vi "Queued Pedestrian Lights.vi"() -> ()   [LabVIEW 2012]
doc: "Traffic Light VI with the use of Queues. Has control over both the Traffic Lights Display and the Pedestrian Lights Display. Red is set as the initial State."
uses:
  Controls/Traffic Light Display.ctl
  Controls/Pedestrian Light Display.ctl
  Controls/Traffic Light States (with Walk State).ctl
panel:
  out "Pedestrian Light Display":T1
  in  "Walk":bool
  in  "Stop Button":bool
  out "Traffic Light Display":T2
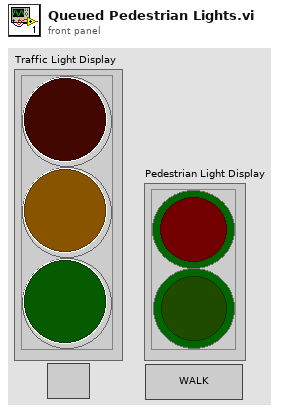
[diagram p1: front panel]
types:
  T1 = typedef "Pedestrian Light Display.ctl" = cluster{"Red":bool, "Green":bool}
  T2 = typedef "Traffic Light Display.ctl" = cluster{"RED":bool, "AMBER":bool, "GREEN":bool}
  T3 = typedef "Traffic Light States (with Walk State).ctl" = enum16{"Red", "RedAmber", "Green", "Amber", "Walk"}
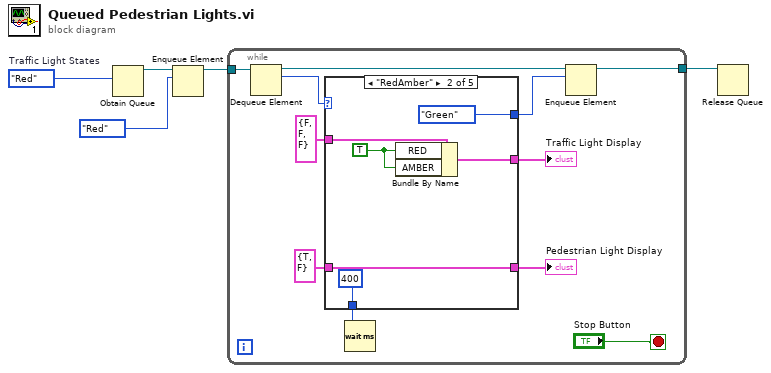
[diagram p0: block diagram]
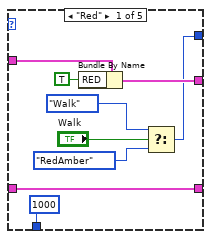
[diagram p2: hidden frame]
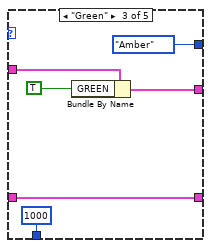
[diagram p3: hidden frame]
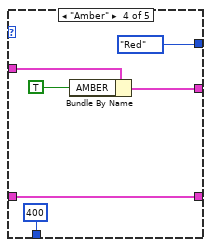
[diagram p4: hidden frame]
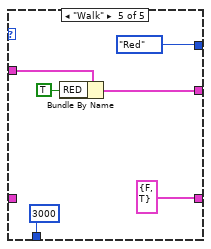
[diagram p5: hidden frame]
diagram:
  w2 = Traffic_Light_States_(with_Walk_State)."Red"  # Traffic Light States
  n1 = Obtain Queue(element data type=w2) -> (queue out=w5:refnum<queue>)  [unwired: 4 in, 2 out]
  n2 = Enqueue Element(queue=w5, element=Traffic_Light_States_(with_Walk_State)."Red") -> (queue out=w4:refnum<queue>)  [unwired: 2 in, 2 out]
  n3 = while {
    tunnel: w4 -> [w10]
    tunnel: [w6] -> w3
    stop <- "Stop Button" stop-if-true
    n4 = Dequeue Element(queue=w10) -> (queue out=w7:refnum<queue>, element=w9:T3)  [unwired: 2 in, 2 out]
    n5 = case shown="\"RedAmber\"" w9 {
      tunnel: T2 {"RED"=FALSE, "AMBER"=FALSE, "GREEN"=FALSE} ("Traffic Light Display") -> [w25 w31 w37 w43 w48]
      tunnel: [w23 w30 w35 w41 w46] -> w15
      tunnel: [w20 Traffic_Light_States_(with_Walk_State)."Green" Traffic_Light_States_(with_Walk_State)."Amber" Traffic_Light_States_(with_Walk_State)."Red" Traffic_Light_States_(with_Walk_State)."Red"] -> w8
      tunnel: [1000 400 1000 400 3000] -> w13
      tunnel: T1 {"Red"=TRUE, "Green"=FALSE} ("Pedestrian Light Display") -> [w19 w27 w33 w39 _]
      tunnel: [w19 w27 w33 w39 T1 {"Red"=FALSE, "Green"=TRUE} ("Pedestrian Light Display")] -> w11
      frame "Red" {
        n6 = Bundle By Name(cluster=w25, "RED"=TRUE) -> (w23:T2)
        n7 = Select(t=Traffic_Light_States_(with_Walk_State)."Walk", s="Walk", f=Traffic_Light_States_(with_Walk_State)."RedAmber") -> (s? t:f=w20:T3)
      }
      frame "RedAmber" {
        w29 = TRUE ("RED")
        n8 = Bundle By Name(cluster=w31, "RED"=w29, "AMBER"=w29) -> (w30:T2)
      }
      frame "Green" {
        n9 = Bundle By Name(cluster=w37, "GREEN"=TRUE ("RED")) -> (w35:T2)
      }
      frame "Amber" {
        n10 = Bundle By Name(cluster=w43, "AMBER"=TRUE ("RED")) -> (w41:T2)
      }
      frame "Walk" {
        n11 = Bundle By Name(cluster=w48, "RED"=TRUE) -> (w46:T2)
      }
    }
    "Traffic Light Display" <- w15
    "Pedestrian Light Display" <- w11
    n12 = Wait (ms)(milliseconds to wait=w13) -> ()  [unwired: 1 out]
    n13 = Enqueue Element(queue=w7, element=w8) -> (queue out=w6:refnum<queue>)  [unwired: 2 in, 2 out]
  }
  n14 = Release Queue(queue=w3) -> ()  [unwired: 2 in, 3 out]
